vi "QDMH Error Dialog.vi"(8 "error":errorcluster, 11 "Case Error Occured":string) -> (0 "error out (no error)":errorcluster, 3 "Case to Execute":string)   [LabVIEW 2019]
doc: "This VI will display a dialog box to the user in the instance of a non filtered error. The user has the option to continue or exit. Additionally it lets the user know which case caused the error.\n\nAAL 9/09"
uses:
  <vilib>/Utility/error.llb/DialogType.ctl
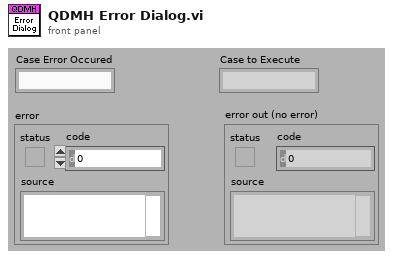
[diagram p1: front panel]
types:
  T1 = typedef "DialogType.ctl" = u16
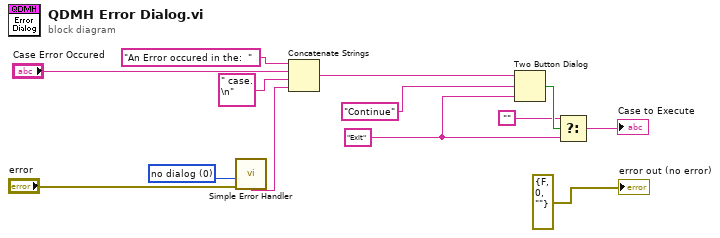
[diagram p0: block diagram]
diagram:
  w2 = "Exit" ("F button name (\"Cancel\")")
  w4 = T1 0 items=["no dialog", "OK message", "continue or stop message", "OK message + warnings", "continue/stop + warnings"] ("type of dialog (OK msg:1)")
  n1 = call <vilib>:"Simple Error Handler.vi"("type of dialog (OK msg:1)"=w4, "error in (no error)"="error") -> ("message"=w8:string)  [unwired: 7 out]
  n2 = Concatenate Strings("An Error occured in the:  " ("string"), "Case Error Occured", " case.\n" ("string"), w8) -> (w10:string)
  n3 = Two Button Dialog(message=w10, 1:w2, 2:"Continue" ("T button name (\"OK\")")) -> (T button?=w12:bool)
  n4 = Select(t="", s=w12, f=w2) -> (s? t:f=→"Case to Execute":string)
  "error out (no error)" <- errorcluster {"status"=FALSE, "code"=0, "source"=""} ("error")
